vi "MotherboardTest - TestStand - Initialize Termination Monitor.vi"(8 "error in (no error)":errorcluster, 11 "Sequence Context In":refnum<k7>) -> (0 "error out":errorcluster, 3 "Status Monitor Out":T1)   [LabVIEW 2013]
doc: "Creates the termination monitor data property and execution objects the TestStand - Get Termination Monitor Status VI uses. Use the TestStand - Close Termination Monitor VI to release the termination monitor data property and execution objects."
uses:
  MotherboardTest - TestStand - Status Monitor.ctl
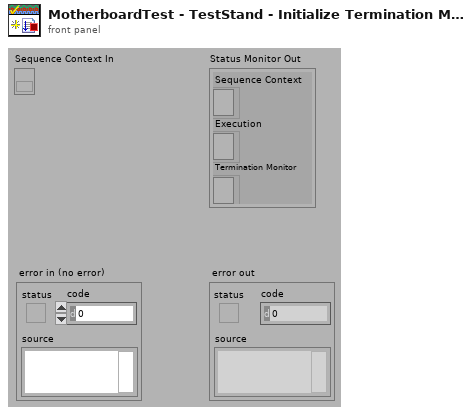
[diagram p1: front panel]
types:
  T1 = typedef "MotherboardTest - TestStand - Status Monitor.ctl" = cluster{"Sequence Context":refnum<k7>, "Execution":refnum<k7>, "Termination Monitor":refnum<k7>}
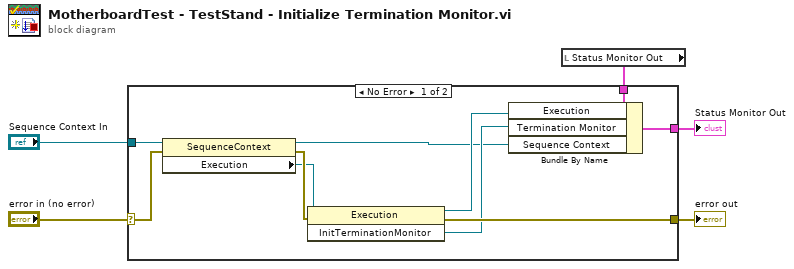
[diagram p0: block diagram]
diagram:
  n1 = local read "Status Monitor Out"() -> (w2:T1)
  n2 = case shown="No Error" "error in (no error)" {
    selector: "error in (no error)" -> [w6 w16]
    tunnel: [w13 w16] -> w5
    tunnel: "Sequence Context In" -> [w12 _]
    tunnel: [w8 w17] -> w3
    tunnel: w2 -> [w7 w17]
    frame No Error {
      n3 = property class="SequenceContext"(reference=w12, error in=w6) -> (reference out=w9:refnum<k7>, error out=w15:errorcluster, "Execution"=w14:refnum<k7>)
      n4 = invoke class="Execution" method="InitTerminationMonitor"(reference=w14, error in=w15) -> (reference out=w11:refnum<k7>, error out=w13:errorcluster, "InitTerminationMonitor"=w10:refnum<k7>)  [unwired: 1 in]
      n5 = Bundle By Name(cluster=w7, "Execution"=w11, "Termination Monitor"=w10, "Sequence Context"=w9) -> (w8:T1)
    }
    frame Error {
    }
  }
  "Status Monitor Out" <- w3
  "error out" <- w5
